vi "Counter - Finite Output.vi"() -> ()   [LabVIEW 2020]
doc: "This example demonstrates how to generate a finite number of digital pulses using a counter output.\n\nOn some hardware, this requires the use of a second counter to generate a gate signal. If necessary, DAQmx configures this second counter for you."
uses:
  <vilib>/DAQmx/write.llb/DAQmx Write (Analog Wfm 1Chan NSamp).vi
  <vilib>/Utility/file.llb/Read Delimited Spreadsheet (DBL).vi
  <vilib>/DAQmx/create/channels.llb/DAQmx Create Channel (AO-Voltage-Basic).vi
  <vilib>/DAQmx/configure/timing.llb/DAQmx Timing (Sample Clock).vi
  <vilib>/DAQmx/miscellaneous.llb/DAQmx Fill In Error Info.vi
  Global stop DAQ.vi
  <vilib>/DAQmx/create/channels.llb/DAQmx Create Channel (CO-Pulse Generation-Frequency).vi
  <vilib>/DAQmx/configure/timing.llb/DAQmx Timing (Implicit).vi
  Global DAQ started.vi
  <resource>/objmgr/daqmx.rc
  <vilib>/DAQmx/configure/trigger.llb/DAQmx Start Trigger (Digital Edge).vi
  <vilib>/Utility/error.llb/DialogType.ctl
panel:
  in  "initial delay":dbl format="%.6f"
  in  "Number of images":i32=1000
  in  "Setup 2":enum16{"Test setup", "Microscope"}(ring)
  out "actual frequency":dbl=1000.0
  out "CO.Count":u32
  out "task done?":bool
  in  "Setup":enum16{"Test setup", "Microscope"}(ring)
  out "error out 4":errorcluster
  out "error out 3":errorcluster
  in  "stop":bool
  in  "Time Target (s)":dbl=-1.0
  in  "error in":errorcluster
  in  "Delay between frames":dbl=25.0
  in  "Image acquisition time (ms)":dbl=1000.0
  in  "File to read":path=path "C:/Users/lpk27/Documents/pan-ASLMsynched/pan-ASLM/Calibration files/newcalibration_voice coil input_25msflyback.txt"
  out "LabVIEW generated Sawtooth input (blue) and Camera trigger (red)":waveform(dbl)(graph)={"t0"=timestamp(0 s since 1904-01-01), "dt"=1.0, "Y"=array[3075 elements]}
  out "# Samples written per channel":u32=3075
  in  "Number of Pulses":i32=1000
  out "Actual Duty Cycle":dbl
  out "Actual Frequency":dbl
  in  "Duty Cycle":dbl=0.5 format="%.6f"
  in  "Frequency":dbl=1.0 format="%.6f"
  in  "Output Terminal":tag="/Dev1/PFI12"
  in  "Trigger Type":enum32{"No Trigger", "Digital Start"}(tab)
  in  "Retriggerable":bool
  in  "Edge":i32(ring)=10280 items=["Rising"=10280, "Falling"=10171]
  in  "Digital Trigger Source":tag
  in  "Stop":bool
  in  "Counter":tag="Dev1/ctr0"
  # "Channel Settings"
  # "Timing Settings"
  # "Trigger Settings"
  # "To configure and use a trigger you must have the necessary tab selected above."
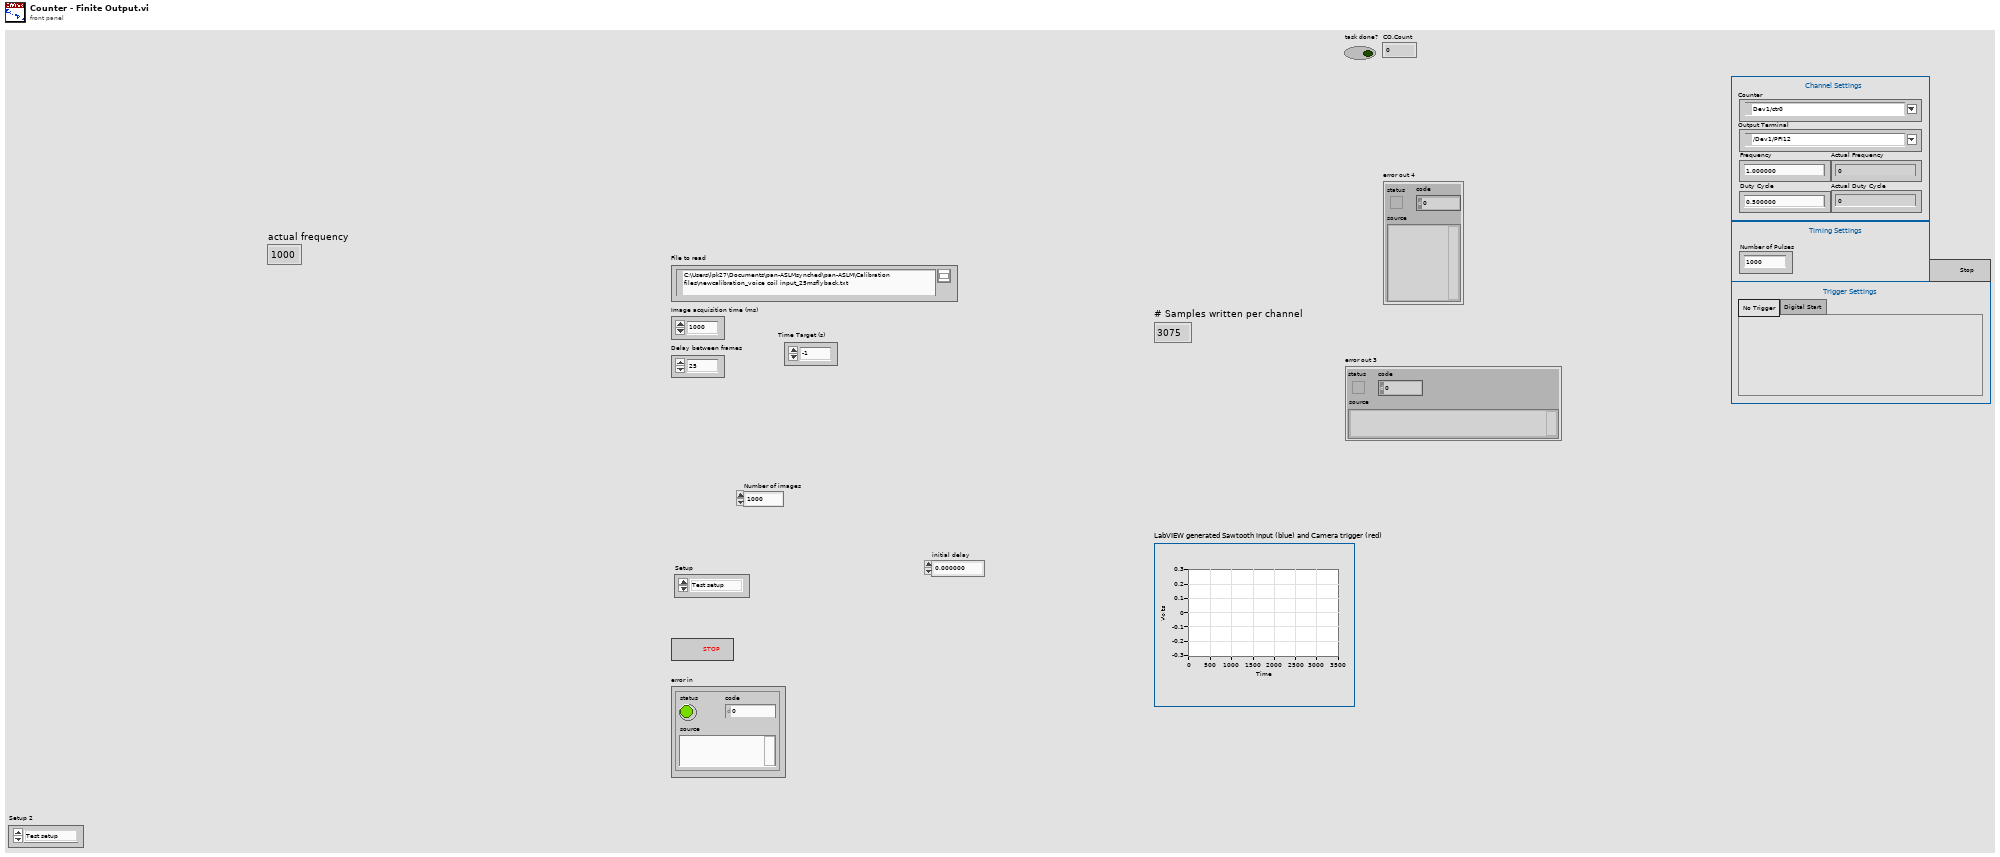
[diagram p1: front panel]
types:
  T1 = typedef "DAQ_channel_typedef.ctl" = cluster{"CO.Pulse.Term":tag, "Voice coil analog output":tag, "counter":tag, "CO.Pulse.Term 2":tag, "AOTF lines":tag, "counter 2":tag, "CO.Pulse.Term 3":tag, "counter 3":tag}
  T2 = typedef "DialogType.ctl" = u16
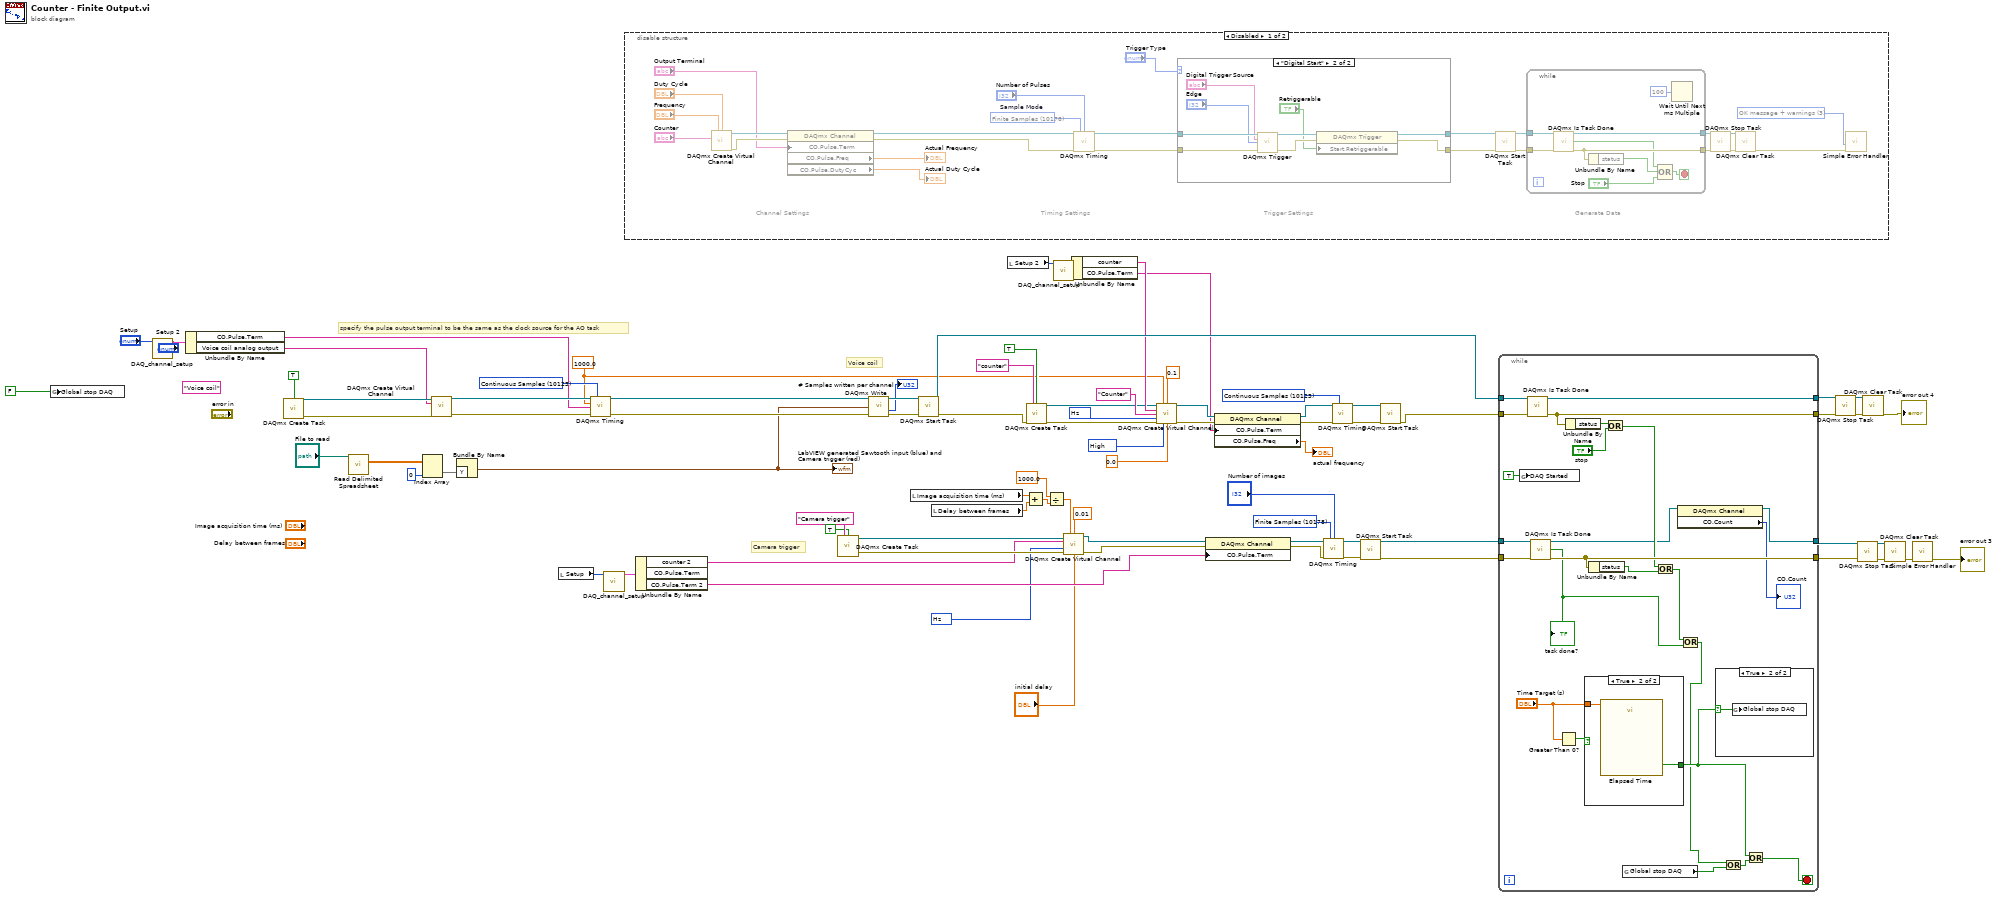
[diagram p0: block diagram]
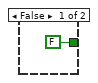
[diagram p5: hidden frame]
diagram:
  w16 = 10192 items=["High"=10192, "Low"=10214] ("idle state")
  w17 = 10373 items=["Hz"=10373] ("units")
  w15 = 10123 items=["Finite Samples"=10178, "Continuous Samples"=10123, "Hardware Timed Single Point"=12522] ("sample mode")
  w34 = 10373 items=["Hz"=10373] ("units")
  (unwired) "Voice coil" ("new task name")
  w71 = 10178 items=["Finite Samples"=10178, "Continuous Samples"=10123, "Hardware Timed Single Point"=12522] ("sample mode")
  w4 = 1000.0 ("rate")
  w81 = 10123 items=["Finite Samples"=10178, "Continuous Samples"=10123, "Hardware Timed Single Point"=12522] ("sample mode")
  # "Voice coil"
  # "Camera trigger"
  # "specify the pulse output terminal to be the same as the clock source for the AO task"
  n1 = global write "Global stop DAQ.vi" "Global stop DAQ"(FALSE ("Global stop DAQ")) -> ()
  n2 = call "DAQ_channel_setup.vi"("Text Ring"="Setup") -> ("DAQ channels OUT"=w42:T1)  [unwired: 10 in]
  n3 = Unbundle By Name(w42) -> ("CO.Pulse.Term"=w27:tag, "Voice coil analog output"=w43:tag)
  n4 = call <vilib>:"DAQmx Create Task.vi"("auto cleanup"=TRUE) -> ("task out"=w60:refnum<k21>, "error out"=w59:errorcluster)  [unwired: 13 in]
  n5 = call-poly <vilib>:"Read Delimited Spreadsheet.vi"("file path (dialog if empty)"="File to read") -> ("all rows"=w67:dbl[][])  [unwired: 9 in, 5 out]
  n6 = Index Array(array=w67, index (col)=0 ("disabled index (col)")) -> (element=w65:dbl[])  [unwired: 1 in]
  n7 = call-poly <vilib>:"DAQmx Create Virtual Channel.vi"("task in"=w60, "physical channels"=w43, "error in"=w59) -> ("task out"=w83:refnum<k21>, "error out"=w82:errorcluster)  [unwired: 11 in]
  n8 = Bundle By Name("Y"=w65) -> (w28:waveform(dbl))  [unwired: 1 in]
  "LabVIEW generated Sawtooth input (blue) and Camera trigger (red)" <- w28
  n9 = local read "Setup"() -> (w38:enum16{"Test setup", "Microscope"})
  n10 = call-poly <vilib>:"DAQmx Timing.vi"("task/channels in"=w83, "sample mode"=w81, "rate"=w4, "source"=w27, "error in"=w82) -> ("task out"=w77:refnum<k21>, "error out"=w76:errorcluster)  [unwired: 9 in]
  n11 = call "DAQ_channel_setup.vi"("Text Ring"=w38) -> ("DAQ channels OUT"=w41:T1)  [unwired: 10 in]
  n12 = disable-structure shown="Disabled" {
    frame Disabled {
      w84 = T2 3 items=["no dialog", "OK message", "continue or stop message", "OK message + warnings", "continue/stop + warnings"] ("type of dialog (OK msg:1)")
      w108 = 10178 items=["Finite Samples"=10178, "Continuous Samples"=10123, "Hardware Timed Single Point"=12522]  # Sample Mode
      # "Generate Data"
      # "Trigger Settings"
      # "Timing Settings"
      # "Channel Settings"
      n13 = call-poly <vilib>:"DAQmx Create Virtual Channel.vi"("frequency"="Frequency", "duty cycle"="Duty Cycle", "counter"="Counter") -> ("task out"=w98:refnum<k21>, "error out"=w97:errorcluster)  [unwired: 11 in]
      n14 = property class="DAQmx Channel"(reference=w98, error in=w97, "CO.Pulse.Term"="Output Terminal") -> (reference out=w94:refnum<k21>, error out=w95:errorcluster, "CO.Pulse.Freq"=→"Actual Frequency":dbl, "CO.Pulse.DutyCyc"=→"Actual Duty Cycle":dbl)
      n15 = call-poly <vilib>:"DAQmx Timing.vi"("task/channels in"=w94, "sample mode"=w108, "samples per channel"="Number of Pulses", "error in"=w95) -> ("task out"=w102:refnum<k21>, "error out"=w101:errorcluster)  [unwired: 10 in]
      n16 = case shown="\"Digital Start\"" "Trigger Type" {
        tunnel: w102 -> [w119 w128]
        tunnel: w101 -> [w118 w127]
        tunnel: [w119 w124] -> w99
        tunnel: [w118 w123] -> w100
        frame "No Trigger", Default {
        }
        frame "Digital Start" {
          n17 = call-poly <vilib>:"DAQmx Trigger.vi"("task/channels in"=w128, "source"="Digital Trigger Source", "edge"="Edge", "error in"=w127) -> ("task out"=w121:refnum<k21>, "error out"=w122:errorcluster)  [unwired: 10 in]
          n18 = property class="DAQmx Trigger"(reference=w121, error in=w122, "Start.Retriggerable"="Retriggerable") -> (reference out=w124:refnum<k21>, error out=w123:errorcluster)
        }
      }
      n19 = call <vilib>:"DAQmx Start Task.vi"("task/channels in"=w99, "error in"=w100) -> ("task out"=w107:refnum<k21>, "error out"=w106:errorcluster)  [unwired: 12 in]
      n20 = while {
        tunnel: w107 -> [w117]
        tunnel: w106 -> [w116]
        tunnel: [w113] -> w85
        tunnel: [w114] -> w86
        stop <- w115 stop-if-true
        n21 = call <vilib>:"DAQmx Is Task Done.vi"("task/channels in"=w117, "error in"=w116) -> ("task out"=w114:refnum<k21>, "task done?"=w109:bool, "error out"=w113:errorcluster)  [unwired: 11 in]
        n22 = Unbundle By Name(w113) -> ("status"=w112:bool)
        n23 = Compound Arithmetic op=OR(w109, w112, "Stop") -> (w115:bool)
        n24 = Wait Until Next ms Multiple(millisecond multiple=u32 100) -> ()  [unwired: 1 out]
      }
      n25 = call <vilib>:"DAQmx Stop Task.vi"("task/channels in"=w86, "error in"=w85) -> ("task out"=w88:refnum<k21>, "error out"=w87:errorcluster)  [unwired: 12 in]
      n26 = call <vilib>:"DAQmx Clear Task.vi"("task in"=w88, "error in"=w87) -> ("error out"=w105:errorcluster)  [unwired: 13 in]
      n27 = call <vilib>:"Simple Error Handler.vi"("type of dialog (OK msg:1)"=w84, "error in (no error)"=w105) -> ()  [unwired: 3 in, 5 out]
    }
    frame Enabled {
    }
  }
  n28 = Unbundle By Name(w41) -> ("counter 2"=w40:tag, "CO.Pulse.Term 2"=w35:tag)  [unwired: 1 out]
  n29 = call <vilib>:"DAQmx Create Task.vi"("new task name"="Camera trigger", "auto cleanup"=TRUE) -> ("task out"=w56:refnum<k21>, "error out"=w57:errorcluster)  [unwired: 12 in]
  n30 = call-poly <vilib>:"DAQmx Write.vi"("task/channels in"=w77, "data"=w28, "error in"=w76) -> ("task out"=w80:refnum<k21>, "number of samples written per channel"=→"# Samples written per channel":u32, "error out"=w79:errorcluster)  [unwired: 10 in]
  n31 = local read "Image acquisition time (ms)"() -> (w62:dbl)
  n32 = call <vilib>:"DAQmx Start Task.vi"("task/channels in"=w80, "error in"=w79) -> ("task out"=w36:refnum<k21>, "error out"=w5:errorcluster)  [unwired: 12 in]
  n33 = local read "Delay between frames"() -> (w61:dbl)
  n34 = local read "Setup 2"() -> (w11:enum16{"Test setup", "Microscope"})
  n35 = Add(x=w62, y=w61) -> (x+y=w30:dbl)
  n36 = call <vilib>:"DAQmx Create Task.vi"("new task name"="counter", "auto cleanup"=TRUE, "error in"=w5) -> ("task out"=w8:refnum<k21>, "error out"=w24:errorcluster)  [unwired: 11 in]
  n37 = Divide(x=1000.0 ("y"), y=w30) -> (x/y=w33:dbl)
  n38 = call "DAQ_channel_setup.vi"("Text Ring"=w11) -> ("DAQ channels OUT"=w13:T1)  [unwired: 10 in]
  n39 = call-poly <vilib>:"DAQmx Create Virtual Channel.vi"("task in"=w56, "frequency"=w33, "duty cycle"=0.01, "counter"=w40, "units"=w34, "error in"=w57, "initial delay"="initial delay") -> ("task out"=w75:refnum<k21>, "error out"=w64:errorcluster)  [unwired: 7 in]
  n40 = Unbundle By Name(w13) -> ("counter"=w12:tag, "CO.Pulse.Term"=w3:tag)
  n41 = call-poly <vilib>:"DAQmx Create Virtual Channel.vi"("task in"=w8, "frequency"=w4, "duty cycle"=0.1, "counter"=w12, "name to assign"="Counter", "units"=w17, "error in"=w24, "idle state"=w16, "initial delay"=0.0) -> ("task out"=w23:refnum<k21>, "error out"=w22:errorcluster)  [unwired: 5 in]
  n42 = property class="DAQmx Channel"(reference=w75, error in=w64, "CO.Pulse.Term"=w35) -> (reference out=w63:refnum<k21>, error out=w72:errorcluster)
  n43 = property class="DAQmx Channel"(reference=w23, error in=w22, "CO.Pulse.Term"=w3) -> (reference out=w20:refnum<k21>, error out=w21:errorcluster, "CO.Pulse.Freq"=→"actual frequency":dbl)
  n44 = call-poly <vilib>:"DAQmx Timing.vi"("task/channels in"=w63, "sample mode"=w71, "samples per channel"="Number of images", "error in"=w72) -> ("task out"=w70:refnum<k21>, "error out"=w69:errorcluster)  [unwired: 10 in]
  n45 = call-poly <vilib>:"DAQmx Timing.vi"("task/channels in"=w20, "sample mode"=w15, "error in"=w21) -> ("task out"=w26:refnum<k21>, "error out"=w25:errorcluster)  [unwired: 11 in]
  n46 = call <vilib>:"DAQmx Start Task.vi"("task/channels in"=w70, "error in"=w69) -> ("task out"=w74:refnum<k21>, "error out"=w73:errorcluster)  [unwired: 12 in]
  n47 = call <vilib>:"DAQmx Start Task.vi"("task/channels in"=w26, "error in"=w25) -> ("error out"=w6:errorcluster)  [unwired: 12 in, 1 out]
  n48 = while {
    tunnel: w36 -> [w152]
    tunnel: w74 -> [w151]
    tunnel: w73 -> [w150]
    tunnel: [w149] -> w45
    tunnel: [w147] -> w44
    tunnel: [w131] -> w49
    tunnel: [w148] -> w48
    tunnel: w6 -> [w129]
    stop <- w140 stop-if-true
    n49 = global write "Global DAQ started.vi" "DAQ Started"(TRUE ("DAQ Started")) -> ()
    n50 = call <vilib>:"DAQmx Is Task Done.vi"("task/channels in"=w152, "error in"=w129) -> ("task out"=w149:refnum<k21>, "error out"=w147:errorcluster)  [unwired: 11 in, 1 out]
    n51 = call <vilib>:"DAQmx Is Task Done.vi"("task/channels in"=w151, "error in"=w150) -> ("task out"=w132:refnum<k21>, "task done?"=w134:bool, "error out"=w148:errorcluster)  [unwired: 11 in]
    "task done?" <- w134
    n52 = Greater Than 0?(x="Time Target (s)") -> (x > 0?=w139:bool)
    n53 = Unbundle By Name(w147) -> ("status"=w144:bool)
    n54 = case shown="True" w139 {
      tunnel: [FALSE ("Time has Elapsed") w156] -> w136
      tunnel: "Time Target (s)" -> [_ w155]
      frame False {
      }
      frame True {
        n55 = call "Elapsed Time"("Time Target (s)"=w155) -> ("Time has Elapsed"=w156:bool)  [unwired: 11 in, 7 out]
      }
    }
    n56 = Unbundle By Name(w148) -> ("status"=w146:bool)
    n57 = Or(x=w144, y="stop") -> (x .or. y?=w142:bool)
    n58 = global read "Global stop DAQ.vi" "Global stop DAQ"() -> (w145:bool)
    n59 = Or(x=w142, y=w146) -> (x .or. y?=w135:bool)
    n60 = property class="DAQmx Channel"(reference=w132) -> (reference out=w131:refnum<k21>, "CO.Count"=→"CO.Count":u32)  [unwired: 1 in, 1 out]
    n61 = Or(x=w135, y=w134) -> (x .or. y?=w133:bool)
    n62 = case shown="True" w136 {
      selector: w136 -> [_ w153]
      frame False {
      }
      frame True {
        n63 = global write "Global stop DAQ.vi" "Global stop DAQ"(w153) -> ()
      }
    }
    n64 = Or(x=w133, y=w145) -> (x .or. y?=w141:bool)
    n65 = Or(x=w136, y=w141) -> (x .or. y?=w140:bool)
  }
  n66 = call <vilib>:"DAQmx Stop Task.vi"("task/channels in"=w45, "error in"=w44) -> ("task out"=w47:refnum<k21>, "error out"=w46:errorcluster)  [unwired: 12 in]
  n67 = call <vilib>:"DAQmx Stop Task.vi"("task/channels in"=w49, "error in"=w48) -> ("task out"=w52:refnum<k21>, "error out"=w53:errorcluster)  [unwired: 12 in]
  n68 = call <vilib>:"DAQmx Clear Task.vi"("task in"=w47, "error in"=w46) -> ("error out"=→"error out 4":errorcluster)  [unwired: 13 in]
  n69 = call <vilib>:"DAQmx Clear Task.vi"("task in"=w52, "error in"=w53) -> ("error out"=w51:errorcluster)  [unwired: 13 in]
  n70 = call <vilib>:"Simple Error Handler.vi"("error in (no error)"=w51) -> ("error out"=→"error out 3":errorcluster)  [unwired: 4 in, 4 out]
